vi "RT Loop - Log Data.vi"(8 "error in (no error)":errorcluster, 9 "Acceleration RT FIFO In":T1, 11 "Message Queue":refnum<queue>) -> ()   [LabVIEW 2017]
doc: "Receive triggered data from Analyze Acceleration Loop and log the data to disk."
uses:
  Globals/Global - All RT Loop Stop.vi
  Globals/Global - Configuration Options.vi
  UI Error Handlers/support/Logging/Logging.lvlib
  UI Error Handlers/support/Message Queue/Message Cluster.ctl
  UI Error Handlers/support/Message Queue/Message Queue.lvlib
  controls/Acceleration RT FIFO Reference.ctl
panel:
  out "AVI Path":path
  out "Acceleration Log Folder":path=path "/home/lvuser/Log/logfiles_deploy"
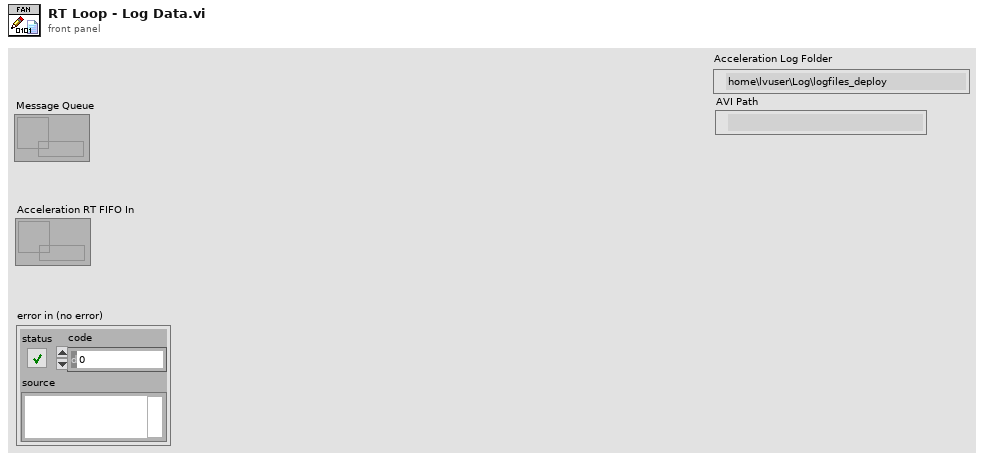
[diagram p1: front panel]
types:
  T1 = typedef "Acceleration RT FIFO Reference.ctl" = refnum<k33>
  T2 = cluster{"Tool data":cluster{"Number of teeth":sgl}, "Cutting data":cluster{"rpm":sgl}, "Limits":cluster{"Magnitude threshold":sgl, "Tolerance":sgl}, "G1 status":cluster{"G1 trigger":bool}}
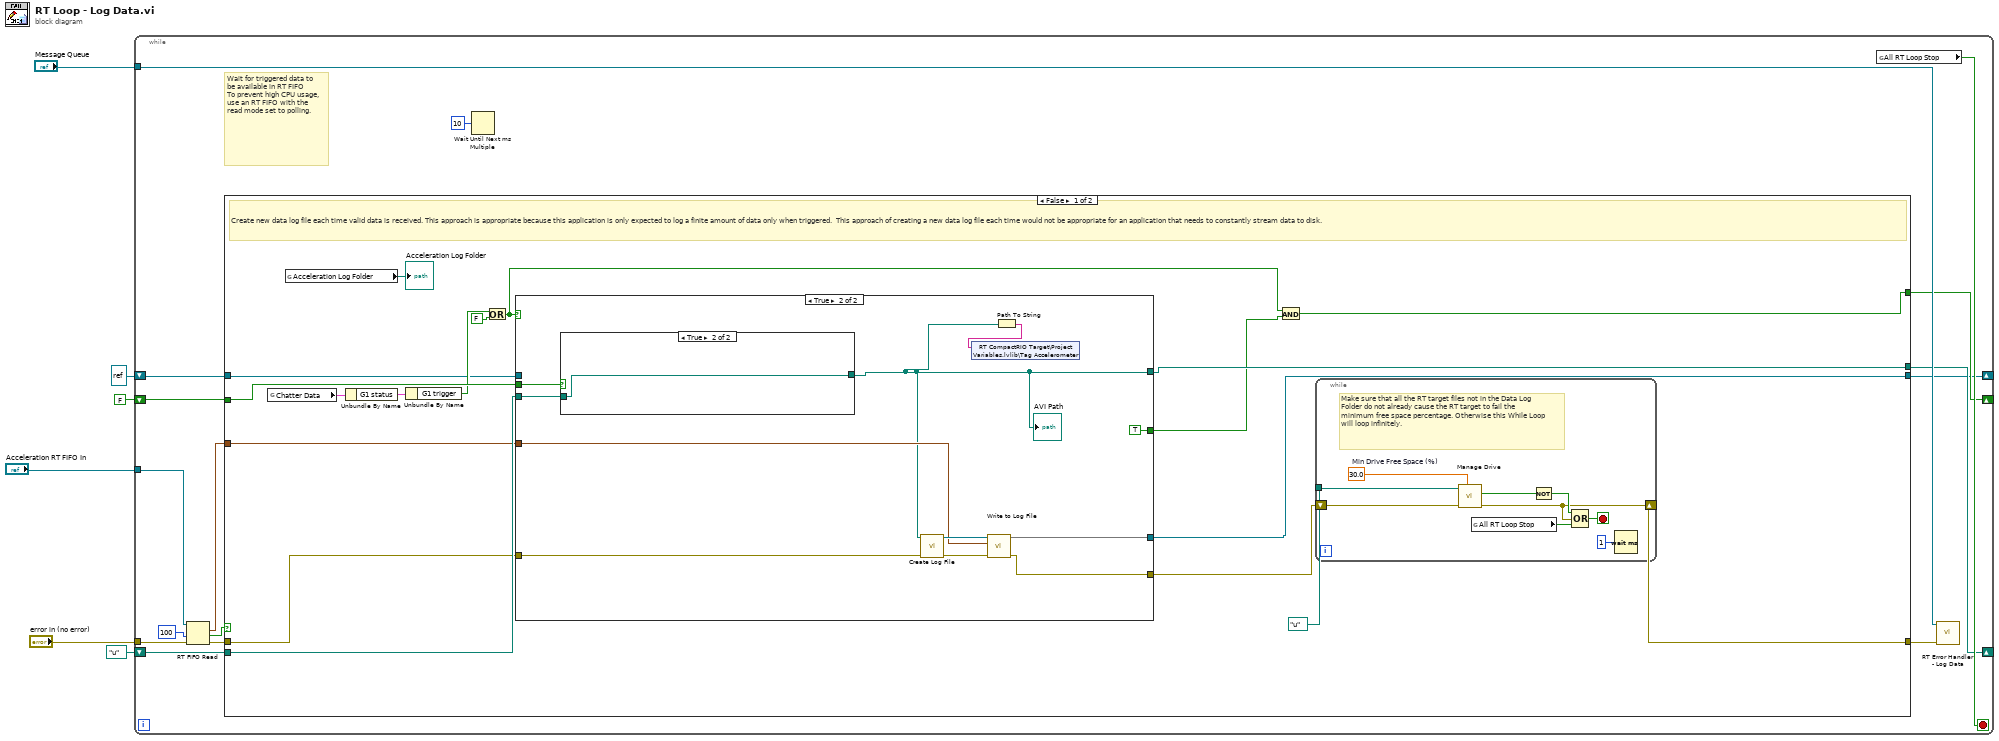
[diagram p0: block diagram]
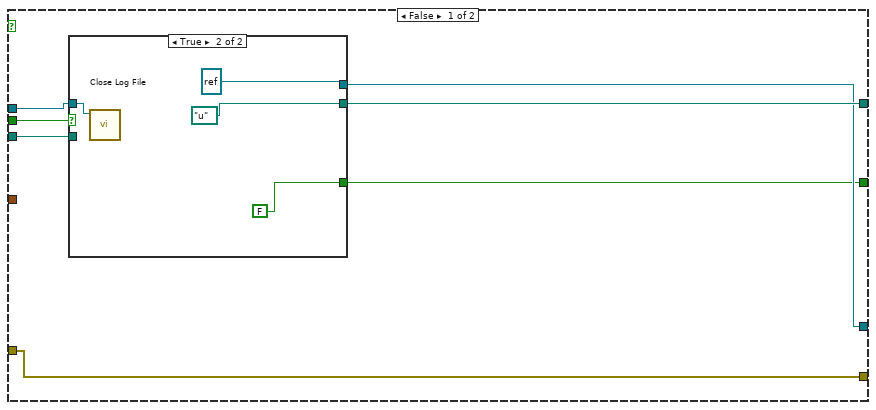
[diagram p2: hidden frame]
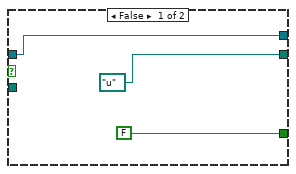
[diagram p3: hidden frame]
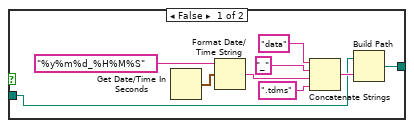
[diagram p4: hidden frame]
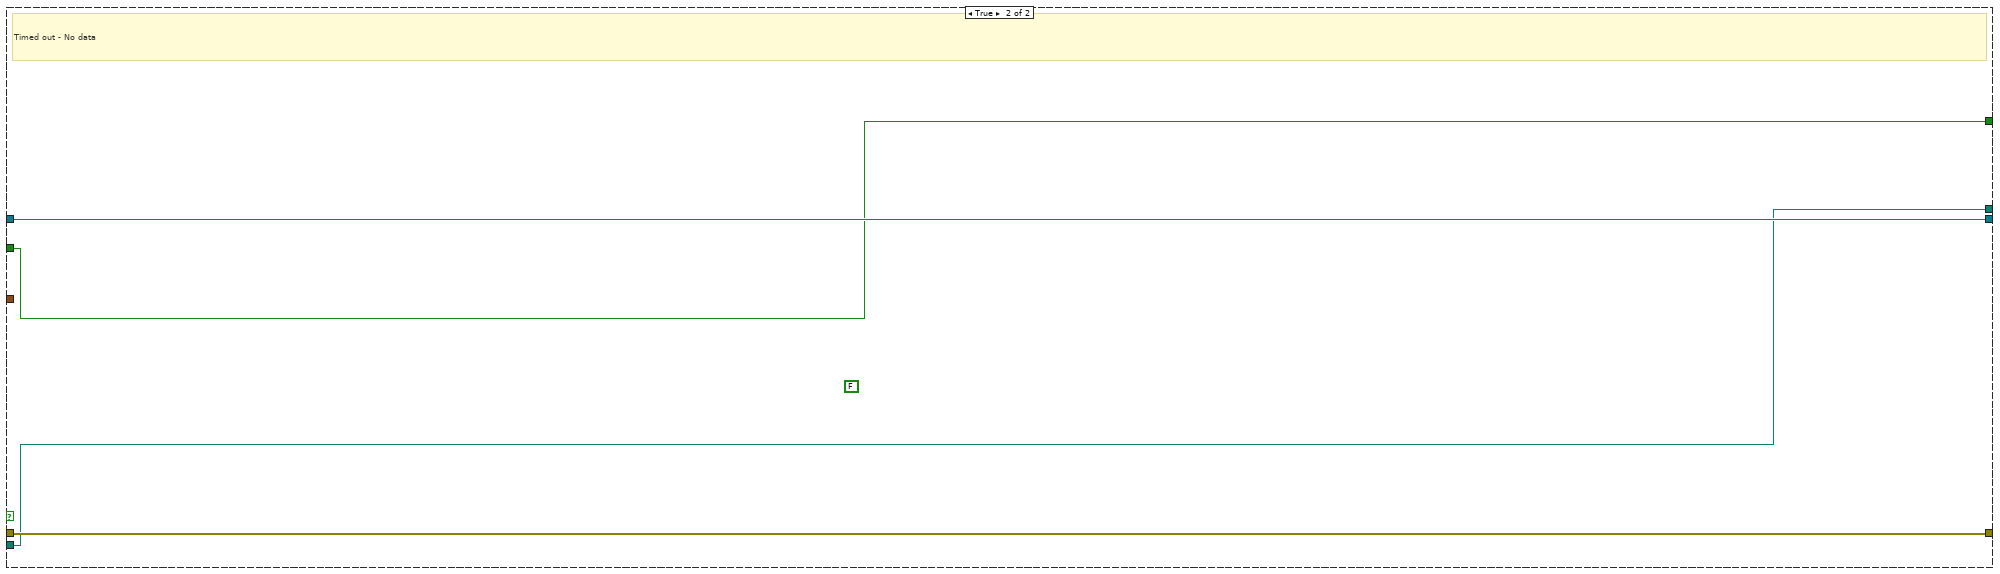
[diagram p5: hidden frame]
diagram:
  n1 = while {
    tunnel: "Acceleration RT FIFO In" -> [w20]
    tunnel: "Message Queue" -> [w17]
    tunnel: "error in (no error)" -> [w22]
    shift-right: [w13] -> _
    shift-left: path "u:/" ("AVI Path") -> [w12]
    shift-right: [w11] -> _
    shift-left: FALSE ("G1 trigger") -> [w10]
    shift-right: [w9] -> _
    shift-left: refnum<k34> refnum ("Log File out") -> [w8]
    stop <- w18 stop-if-true
    # "Wait for triggered data to be available in RT FIFO\nTo prevent high CPU usage, use an RT FIFO with the read mode set to polling."
    n2 = RT FIFO Read(0:w20, 2:100 ("ms timeout (0)"), 3:w22) -> (9:w19:waveform(dbl)[], 10:w14:bool, 11:w21:errorcluster)  [unwired: 1 in, 2 out]
    n3 = case shown="False" w14 {
      tunnel: w19 -> [w30 _]
      tunnel: w21 -> [w28 w88]
      tunnel: [w31 w88] -> w16
      tunnel: [w26 w85] -> w13
      tunnel: w12 -> [w36 w85]
      tunnel: [w23 w86] -> w11
      tunnel: w10 -> [w35 w86]
      tunnel: [w29 w87] -> w9
      tunnel: w8 -> [w32 w87]
      frame False {
        # "Create new data log file each time valid data is received. This approach is appropriate because this application is only expected to log a finite amount of data only when triggered.  This approach of creating a new data log file each time would not be appropriate for an application that needs to constantly stream data to disk."
        n4 = global read "Global - Configuration Options.vi" "Chatter Data"() -> (w38:T2)
        n5 = global read "Global - Configuration Options.vi" "Acceleration Log Folder"() -> (→"Acceleration Log Folder":path)
        n6 = Unbundle By Name(w38) -> ("G1 status"=w37:cluster{"G1 trigger":bool})
        n7 = Unbundle By Name(w37) -> ("G1 trigger"=w34:bool)
        n8 = Or(x=w34, y=FALSE) -> (x .or. y?=w24:bool)
        n9 = case shown="True" w24 {
          tunnel: w36 -> [w44 w65]
          tunnel: [w47 w56] -> w26
          tunnel: w35 -> [w45 w64]
          tunnel: w32 -> [w46 _]
          tunnel: w30 -> [_ w61]
          tunnel: [w43 w59] -> w29
          tunnel: w28 -> [w42 w58]
          tunnel: [w42 w57] -> w27
          tunnel: [w41 TRUE] -> w25
          frame False {
            n10 = case shown="True" w45 {
              tunnel: [path "u:/" ("AVI Path") path "u:/" ("AVI Path")] -> w47
              tunnel: w46 -> [w49 w53]
              tunnel: w44 -> [_ _]
              tunnel: [w49 refnum<k34> refnum ("Log File out")] -> w43
              tunnel: [FALSE FALSE] -> w41
              frame False {
              }
              frame True {
                n11 = call "Close Log File.vi"("tdms file"=w53) -> ()  [unwired: 10 in, 1 out]
              }
            }
          }
          frame True {
            n12 = case shown="True" w64 {
              tunnel: w65 -> [w67 w75]
              tunnel: [w66 w75] -> w56
              frame False {
                n13 = Get Date/Time In Seconds() -> (seconds since 1Jan1904=w70:timestamp)
                n14 = Format Date/Time String(time format string (%c)="%y%m%d_%H%M%S", seconds (now)=w70) -> (date/time string=w73:string)  [unwired: 1 out]
                n15 = Concatenate Strings("data" ("string"), "_" ("string"), w73, ".tdms" ("string")) -> (w68:string)
                n16 = Build Path(base path=w67, name or relative path=w68) -> (appended path=w66:path)
              }
              frame True {
              }
            }
            "AVI Path" <- w56
            n17 = call "Create Log File.vi"("error in (no error)"=w58, "Acceleration Exceeded Log Folder"=w56) -> ("error out"=w63:errorcluster, "Log File out"=w62:refnum<k34>)  [unwired: 8 in]
            n18 = call "Write to Log File.vi"("error in (no error)"=w63, "Array of Waveforms"=w61, "Log File in"=w62) -> ("error out"=w57:errorcluster, 3:w59)  [unwired: 7 in]
            n19 = Path To String(path=w56) -> (string=w60:string)
            n20 = shared-variable "RT CompactRIO Target\\Project Variables.lvlib\\Tag Accelerometer"(w60) -> ()  [unwired: 1 in, 1 out]
          }
        }
        n21 = And(x=w24, y=w25) -> (x .and. y?=w23:bool)
        n22 = while {
          shift-right: [w79] -> w31
          shift-left: w27 -> [w80]
          tunnel: path "u:/" ("AVI Path") -> [w77]
          stop <- w84 stop-if-true
          w78 = 30.0  # Min Drive Free Space (%)
          # "Make sure that all the RT target files not in the Data Log Folder do not already cause the RT target to fail the minimum free space percentage. Otherwise this While Loop will loop infinitely."
          n23 = call "Manage Drive.vi"("Min Drive Free Space (%)"=w78, "error in"=w80, "Data Folder"=w77) -> ("error out"=w79:errorcluster, "Drive Space Below Limit"=w76:bool)  [unwired: 6 in, 1 out]
          n24 = global read "Global - All RT Loop Stop.vi" "All RT Loop Stop"() -> (w81:bool)
          n25 = Not(x=w76) -> (.not. x?=w83:bool)
          n26 = Compound Arithmetic op=OR(w83, w79, w81) -> (w84:bool)
          n27 = Wait (ms)(milliseconds to wait=u32 1) -> ()  [unwired: 1 out]
        }
      }
      frame True {
        (unwired) FALSE
        # "Timed out - No data"
      }
    }
    n28 = Wait Until Next ms Multiple(millisecond multiple=u32 10) -> ()  [unwired: 1 out]
    n29 = global read "Global - All RT Loop Stop.vi" "All RT Loop Stop"() -> (w18:bool)
    n30 = call "RT Error Handler - Log Data.vi"("error in (no error)"=w16, "Message Queue"=w17) -> ()  [unwired: 9 in, 1 out]
  }
